vi "KG number of spumps.vi"(8 "Fehler (Eingang, kein Fehler)":errorcluster, 11 "VISA-Ressourcenname":refnum<visa-resource-name>) -> (0 "Fehler (Ausgang)":errorcluster, 1 "Kommando gesendet":string, 2 "number of spumps":dbl, 3 "VISA-Ressourcenname (Ausgang)":refnum<visa-resource-name>)   [LabVIEW 2020, in "Linearisierung v2.lvlib" / "Gasteiler.lvlib" / "HovaCAL_Interface.lvlib" / "KGN.lvlib" / "get.lvlib"]
uses:
  get.lvlib
  KGN.lvlib
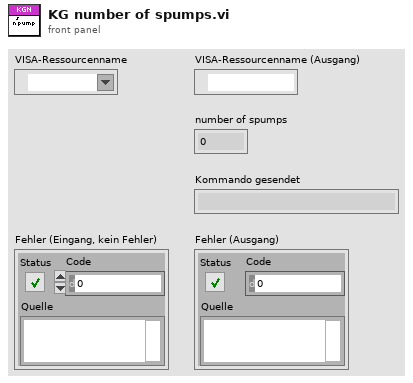
[diagram p1: front panel]
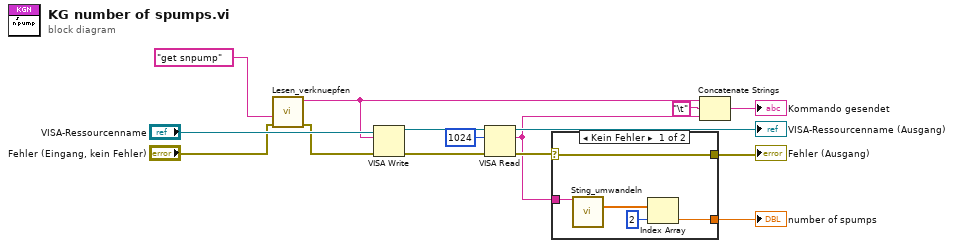
[diagram p0: block diagram]
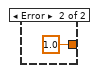
[diagram p2: hidden frame]
diagram:
  n1 = call "Lesen_verknuepfen.vi"("error in (no error)"="Fehler (Eingang, kein Fehler)", "Order"="get snpump" ("Schreibpuffer")) -> ("error out"=w9:errorcluster, "Verknüpfter String"=w2:string)  [unwired: 8 in]
  n2 = VISA Write(VISA resource name="VISA-Ressourcenname", write buffer=w2, error in (no error)=w9) -> (VISA resource name out=w15:refnum<visa-resource-name>, error out=w14:errorcluster)  [unwired: 1 out]
  n3 = VISA Read(VISA resource name=w15, byte count=u32 1024 ("Byte-Anzahl"), error in (no error)=w14) -> (VISA resource name out=→"VISA-Ressourcenname (Ausgang)":refnum<visa-resource-name>, read buffer=w1:string, error out=w7:errorcluster)  [unwired: 1 out]
  n4 = case shown="Kein Fehler" w7 {
    selector: w7 -> [w19 _]
    tunnel: w1 -> [w20 _]
    tunnel: [w16 1.0 ("Zahl 2")] -> w6
    tunnel: [w19 _] -> w5
    frame No Error {
      n5 = call "Sting_umwandeln.vi"("Lesepuffer"=w20) -> ("Zahl array"=w17:dbl[])  [unwired: 8 in, 6 out]
      n6 = Index Array(array=w17, index=2 ("Index")) -> (element=w16:dbl)
    }
    frame Error {
    }
  }
  "Fehler (Ausgang)" <- w5
  "number of spumps" <- w6
  n7 = Concatenate Strings(w2, "\t", w1) -> (→"Kommando gesendet":string)
